vi "Copy_UI_Data.vi"(8 "error in (no error)":errorcluster, 10 "IB_Source in":refnum<class "IB_Source.lvclass">, 11 "IB_TreeContainerItem.lvclass":refnum<class "IB_Tree_Item_Source_Container.lvclass">) -> (0 "error out":errorcluster, 3 "IB_TreeContainerItem out":refnum<class "IB_Tree_Item_Source_Container.lvclass">)   [LabVIEW 2020, in "IB_Tree_Item_Source_Container.lvclass"]
uses:
  <vilib>/AppBuilder/IB_Classes/Tree_Item_Source_Container/IB_Tree_Item_Source_Container.lvclass
  <vilib>/AppBuilder/IB_Classes/Tree_Item_Source_Container/IB_Tree_Item_Source_Container.lvclass/IB_Tree_Item_Source_Container.ctl
  <vilib>/AppBuilder/IB_Classes/Tree_Item_Source_Contained_File/IB_Tree_Item_Source_Contained_File.lvclass
  <vilib>/AppBuilder/IB_Classes/Source/IB_Source.lvclass
  <vilib>/AppBuilder/IB_Classes/Source/Container/IB_Source_Container.lvclass
  <vilib>/AppBuilder/IB_Classes/Tree_Item/IB_Tree_Item.lvclass
  <vilib>/AppBuilder/IB_Classes/Tree_Item_Source/IB_Tree_Item_Source.lvclass
  <vilib>/AppBuilder/IB_Classes/Source/File/CtrFile/IB_CtrFile.lvclass
  <vilib>/AppBuilder/IB_Classes/Tree_Item_Virtual_Folder/IB_Tree_Item_Virtual_Folder.lvclass
  e:/builds/penguin/labview/branches/2020/dev/dist/vi.lib/AppBuilder/IB_Classes/Tree_Item/IB_Tree_Item.lvclass
  e:/builds/penguin/labview/branches/2020/dev/dist/vi.lib/AppBuilder/IB_Classes/Tree_Item_Virtual_Folder/IB_Tree_Item_Virtual_Folder.lvclass
  e:/builds/penguin/labview/branches/2020/dev/dist/vi.lib/AppBuilder/IB_Classes/Tree_Item_Source_File/IB_Tree_Item_Source_File.lvclass
  e:/builds/penguin/labview/branches/2020/dev/dist/vi.lib/AppBuilder/IB_Classes/Tree_Item_Source/IB_Tree_Item_Source.lvclass
  e:/builds/penguin/labview/branches/2020/dev/dist/vi.lib/AppBuilder/IB_Classes/Tree_Item_Source_Contained_File/IB_Tree_Item_Source_Contained_File.lvclass
  e:/builds/penguin/labview/branches/2020/dev/dist/vi.lib/AppBuilder/IB_Classes/Source/IB_Source.lvclass
  e:/builds/penguin/labview/branches/2020/dev/dist/vi.lib/AppBuilder/IB_Classes/Source/Container/IB_Source_Container.lvclass
  e:/builds/penguin/labview/branches/2020/dev/dist/vi.lib/AppBuilder/IB_Classes/Tree_Item_Source_Container/IB_Tree_Item_Source_Container.lvclass
  e:/builds/penguin/labview/branches/2020/dev/dist/vi.lib/AppBuilder/IB_Classes/Source/File/IB_Source_File.lvclass
  e:/builds/penguin/labview/branches/2020/dev/dist/vi.lib/AppBuilder/IB_Classes/Source/File/CtrFile/IB_CtrFile.lvclass
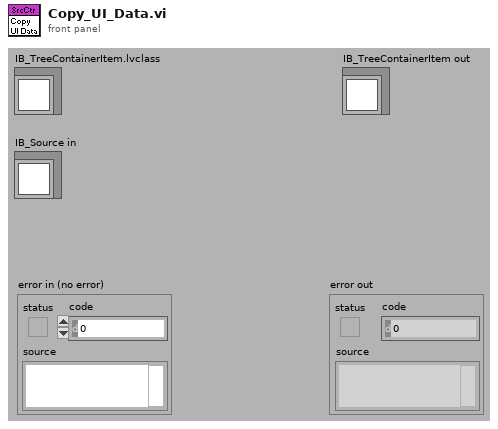
[diagram p1: front panel]
types:
  T1 = typedef "IB_Source_Container.ctl" = cluster{"files":refnum<class "IB_CtrFile.lvclass">[], "previewed?":bool, "preview error?":bool}
  T2 = typedef "IB_Tree_Item.ctl" = cluster{"symbol index":i32, "child tag":string, "parentTag":string, "left cell name":string}
  T3 = typedef "IB_Source.ctl" = cluster{"name":string, "sourceTag":string, "destTag":string, "path":path, "eng_installPath":string, "UI_inBuild?":bool, "str ref?":bool}
  T4 = typedef "IB_Tree_Item_Source_Contained_File.ctl" = cluster{"virt folders":refnum<class "IB_Tree_Item_Virtual_Folder.lvclass">[]}
  T5 = typedef "IB_Tree_Item_Source_Container.ctl" = cluster{"CtrFiles":refnum<class "IB_Tree_Item_Source_Contained_File.lvclass">[]}
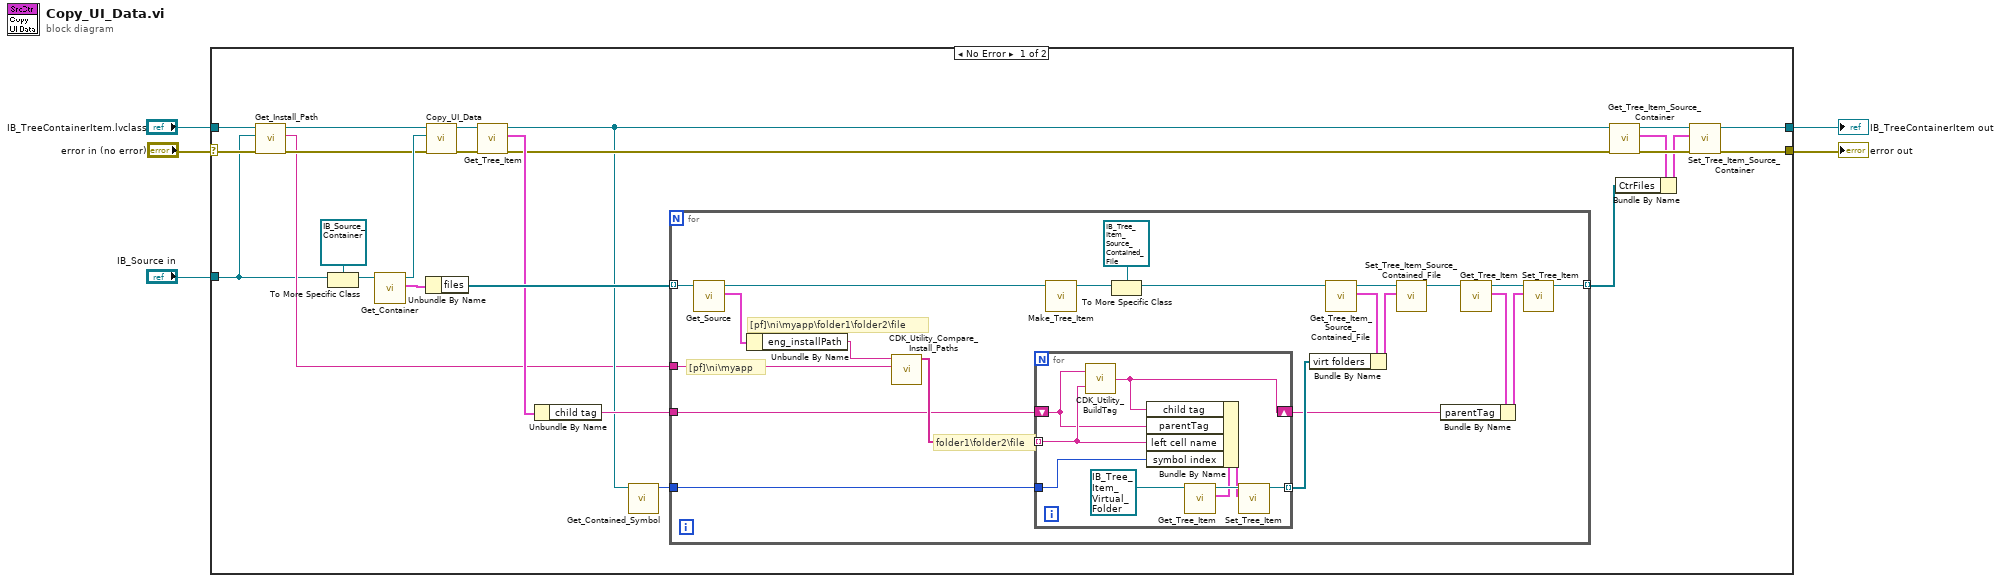
[diagram p0: block diagram]
diagram:
  n1 = case shown="No Error" "error in (no error)" {
    selector: "error in (no error)" -> [w11 w62]
    tunnel: "IB_Source in" -> [w7 _]
    tunnel: "IB_TreeContainerItem.lvclass" -> [w13 w61]
    tunnel: [w17 w61] -> w3
    tunnel: [w16 w62] -> w2
    frame No Error {
      n2 = call-dynamic "Get_Install_Path.vi"("error in (no error)"=w11, "IB_Source in"=w7, "IB_Tree_Item_Source_Container in"=w13) -> ("error out"=w10:errorcluster, "eng_installPath"=w9:string, "IB_Tree_Item_Source_Container out"=w12:refnum<class "IB_Tree_Item_Source_Container.lvclass">)  [unwired: 6 out]
      n3 = To More Specific Class(target class=refnum<class "IB_Source_Container.lvclass"> refnum ("IB_Source_Container.lvclass"), reference=w7) -> (specific class reference=w6:refnum<class "IB_Source_Container.lvclass">)  [unwired: 1 in, 1 out]
      n4 = call <vilib>:"Get_Container.vi"("IB_Source_Container in"=w6) -> ("data"=w30:T1, "IB_Source_Container out"=w23:refnum<class "IB_Source_Container.lvclass">)  [unwired: 1 in, 8 out]
      n5 = Unbundle By Name(w30) -> ("files"=w29:refnum<class "IB_CtrFile.lvclass">[])
      n6 = call-parent "Copy_UI_Data.vi"("error in (no error)"=w10, "IB_Source in"=w23, "IB_TreeSrcItem.lvclass"=w12) -> ("error out"=w21:errorcluster, "IB_TreeSrcItem out"=w22:refnum<class "IB_Tree_Item_Source_Container.lvclass">)  [unwired: 7 out]
      n7 = call <vilib>:"Get_Tree_Item.vi"("error in (no error)"=w21, "IB_TreeItem in"=w22) -> ("error out"=w18:errorcluster, "data"=w20:T2, "IB_TreeItem out"=w14:refnum<class "IB_Tree_Item_Source_Container.lvclass">)  [unwired: 7 out]
      n8 = Unbundle By Name(w20) -> ("child tag"=w19:string)
      n9 = call-dynamic "Get_Contained_Symbol.vi"("IB_Tree_Item_Source_Container in"=w14) -> ("symbol index"=w15:i32)  [unwired: 1 in, 9 out]
      n10 = for {
        tunnel: w29 -> [w48] mode=indexing
        tunnel: [w33] -> w24 mode=indexing
        tunnel: w9 -> [w45]
        tunnel: w19 -> [w43]
        tunnel: w15 -> [w31]
        # "folder1\\folder2\\file"
        # "[pf]\\ni\\myapp"
        # "[pf]\\ni\\myapp\\folder1\\folder2\\file"
        n11 = call <vilib>:"Get_Source.vi"("IB_Source in"=w48) -> ("data"=w46:T3, "IB_Source out"=w47:refnum<class "IB_CtrFile.lvclass">)  [unwired: 1 in, 8 out]
        n12 = Unbundle By Name(w46) -> ("eng_installPath"=w49:string)
        n13 = call <resource>:"CDK_Utility_Compare_Install_Paths.vi"("short"=w45, "long"=w49) -> ("relative path"=w44:string[])  [unwired: 9 out]
        n14 = for {
          tunnel: w44 -> [w58] mode=indexing
          shift-right: [w56] -> w32
          shift-left: w43 -> [w57]
          tunnel: [w54] -> w38 mode=indexing
          tunnel: w31 -> [w53]
          n15 = call <resource>:"CDK_Utility_BuildTag.vi"("name or relative path"=w58, "BasePath"=w57) -> ("appended path"=w56:string)
          n16 = call <vilib>:"Get_Tree_Item.vi"("IB_TreeItem in"=refnum<class "IB_Tree_Item_Virtual_Folder.lvclass"> refnum ("IB_Tree_Item_Virtual_Folder.lvclass")) -> ("data"=w59:T2, "IB_TreeItem out"=w60:refnum<class "IB_Tree_Item_Virtual_Folder.lvclass">)  [unwired: 1 in, 8 out]
          n17 = Bundle By Name(cluster=w59, "child tag"=w56, "parentTag"=w57, "left cell name"=w58, "symbol index"=w53) -> (w55:T2)
          n18 = call <vilib>:"Set_Tree_Item.vi"("data"=w55, "IB_TreeItem in"=w60) -> ("IB_TreeItem out"=w54:refnum<class "IB_Tree_Item_Virtual_Folder.lvclass">)  [unwired: 1 in, 8 out]
        }
        n19 = call-dynamic "Make_Tree_Item.vi"("IB_CtrFile in"=w47) -> ("TreeSrcItem"=w50:refnum<class "IB_Tree_Item_Source.lvclass">)  [unwired: 1 in, 9 out]
        n20 = To More Specific Class(target class=refnum<class "IB_Tree_Item_Source_Contained_File.lvclass"> refnum ("IB_TreeCtrFileItem.lvclass"), reference=w50) -> (specific class reference=w42:refnum<class "IB_Tree_Item_Source_Contained_File.lvclass">)  [unwired: 1 in, 1 out]
        n21 = call <vilib>:"Get_Tree_Item_Source_Contained_File.vi"("IB_TreeCtrFileItem in"=w42) -> ("data"=w40:T4, "IB_TreeCtrFileItem out"=w41:refnum<class "IB_Tree_Item_Source_Contained_File.lvclass">)  [unwired: 1 in, 8 out]
        n22 = Bundle By Name(cluster=w40, "virt folders"=w38) -> (w39:T4)
        n23 = call <vilib>:"Set_Tree_Item_Source_Contained_File.vi"("data"=w39, "IB_TreeCtrFileItem in"=w41) -> ("IB_TreeCtrFileItem out"=w34:refnum<class "IB_Tree_Item_Source_Contained_File.lvclass">)  [unwired: 1 in, 8 out]
        n24 = call <vilib>:"Get_Tree_Item.vi"("IB_TreeItem in"=w34) -> ("data"=w36:T2, "IB_TreeItem out"=w37:refnum<class "IB_Tree_Item_Source_Contained_File.lvclass">)  [unwired: 1 in, 8 out]
        n25 = Bundle By Name(cluster=w36, "parentTag"=w32) -> (w35:T2)
        n26 = call <vilib>:"Set_Tree_Item.vi"("data"=w35, "IB_TreeItem in"=w37) -> ("IB_TreeItem out"=w33:refnum<class "IB_Tree_Item_Source_Contained_File.lvclass">)  [unwired: 1 in, 8 out]
      }
      n27 = call <vilib>:"Get_Tree_Item_Source_Container.vi"("error in (no error)"=w18, "IB_TreeContainerItem in"=w14) -> ("error out"=w27:errorcluster, "data"=w26:T5, "IB_TreeContainerItem out"=w28:refnum<class "IB_Tree_Item_Source_Container.lvclass">)  [unwired: 7 out]
      n28 = Bundle By Name(cluster=w26, "CtrFiles"=w24) -> (w25:T5)
      n29 = call <vilib>:"Set_Tree_Item_Source_Container.vi"("error in (no error)"=w27, "data"=w25, "IB_TreeContainerItem in"=w28) -> ("error out"=w16:errorcluster, "IB_TreeContainerItem out"=w17:refnum<class "IB_Tree_Item_Source_Container.lvclass">)  [unwired: 7 out]
    }
    frame Error {
    }
  }
  "IB_TreeContainerItem out" <- w3
  "error out" <- w2
